vi "Get Database Manager.vi"(8 "error in (no error)":errorcluster, 11 "Parent Child in":refnum<class "Parent Child.lvclass">) -> (0 "error out":errorcluster, 2 "Database Manager":refnum<class "Database Manager.lvclass">, 3 "Parent Child out":refnum<class "Parent Child.lvclass">)   [LabVIEW 2019, in "HierDAL Library.lvlib" / "Database.lvlib" / "Repositories.lvlib" / "Parent Child.lvclass"]
uses:
  Parent Child.lvclass
  Database Manager Class/Database Manager.lvclass
  Parent Child.lvclass/Parent Child.ctl
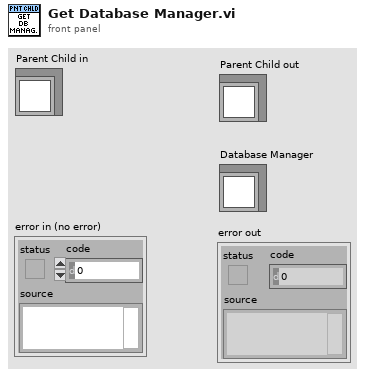
[diagram p1: front panel]
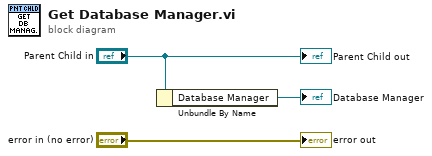
[diagram p0: block diagram]
diagram:
  n1 = Unbundle By Name("Parent Child in") -> ("Database Manager"=→"Database Manager":refnum<class "Database Manager.lvclass">)
  "error out" <- "error in (no error)"
  "Parent Child out" <- "Parent Child in"
